vi "launcher.vi"() -> ()   [LabVIEW 2015, in "lv-interface-re.lvlib"]
uses:
  lv-interface-re.lvlib
  main.vi
panel:
  out "error":errorcluster
  in  "launch":bool
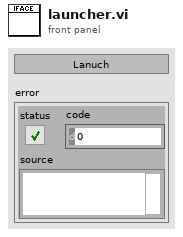
[diagram p1: front panel]
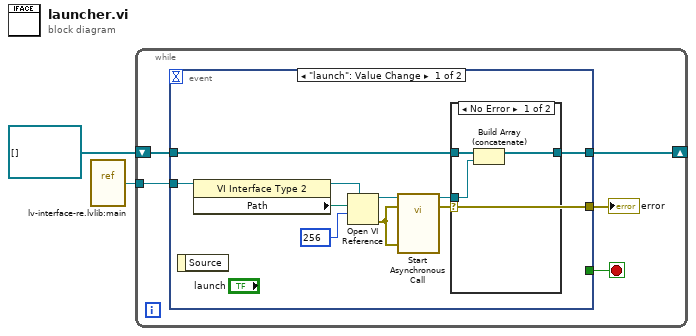
[diagram p0: block diagram]
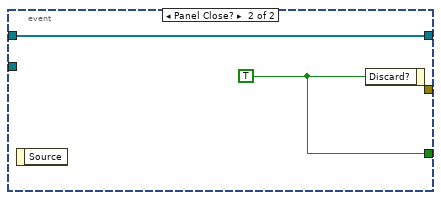
[diagram p3: hidden frame]
diagram:
  n1 = vi-ref "lv-interface-re.lvlib:main.vi"() -> (w1:refnum<vi>)
  n2 = while {
    shift-right: [w5] -> _
    shift-left: refnum<vi>[] [] ("appended array") -> [w6]
    tunnel: w1 -> [w4]
    stop <- w7 stop-if-true
    n3 = event shown="[0] \"launch\": Value Change" {
      selector: _ -> [_ _]
      dyn-events: _ -> [_ _]
      timeout: _ -> [_ _]
      tunnel: [_ w23] -> w7
      tunnel: w6 -> [w12 w22]
      tunnel: [w11 w22] -> w5
      tunnel: w4 -> [w17 _]
      tunnel: [w8 _] -> w3
      event "launch": Value Change {
        n4 = event-data() -> ()  [unwired: 1 in, 1 out]
        n5 = property class="VI Interface Type 2"(reference=w17) -> (reference out=w15:refnum<vi>, "Path"=w16:path)  [unwired: 1 in, 1 out]
        n6 = Open VI Reference(type specifier VI Refnum (for type only)=w15, vi path=w16, options=256) -> (vi reference=w14:refnum<vi>, error out=w13:errorcluster)  [unwired: 3 in]
        n7 = call-by-ref "Start Asynchronous Call"(reference=w14, error in=w13, 8:"error in (no error)"=w13) -> (reference out=w10:refnum<vi>, error out=w8:errorcluster)  [unwired: 10 in, 1 out]
        n8 = case shown="No Error" w8 {
          tunnel: w12 -> [w20 w21]
          tunnel: [w18 w21] -> w11
          tunnel: w10 -> [w19 _]
          frame No Error {
            n9 = Build Array (concatenate)(w20, w19) -> (w18:refnum<vi>[])
          }
          frame Error {
          }
        }
      }
      event Panel Close? {
        w23 = TRUE ("Discard?")
        n10 = event-data() -> ()  [unwired: 1 in, 1 out]
        n11 = event-data("Discard?"=w23) -> ()  [unwired: 1 in, 1 out]
      }
    }
    "error" <- w3
  }
